vi "Consumer.vi"(8 "error in (no error)":errorcluster, 9 "Data":variant, 10 "Case ID":string, 11 "uService Template in":refnum<class "Father of all uServices.lvclass">) -> (0 "error out":errorcluster, 3 "uService Template out":refnum<class "Father of all uServices.lvclass">)   [LabVIEW 2026, in "TALOS.lvlib" / "Father of all uServices.lvlib" / "Father of all uServices.lvclass"]
uses:
  Father of all uServices.lvclass
  Father of all uServices.lvclass/Father of all uServices.ctl
  Ancestor/Ancestor/Ancestor.lvclass/Ancestor.ctl
  Classes/Log/Log.lvclass/Log.ctl
  45abb896-52c1-49c5-8199-1eb3a3dabe5e.vi
  <vilib>/AdvancedString/1D String Array to Delimited String (string).vi
  <vilib>/AdvancedString/Delimited String to 1D String Array.vi
  <vilib>/AdvancedString/Delimited String to 1D String Array (string).vi
  Support VIs/Generate Error.vi
  Classes/Log/Write.vi
  FGV/Error Memory/Get Error Description.vi
  Support VIs/Get PC name.vi
  Ancestor/Ancestor/Read ID.vi
  Support VIs/Date n Time.vi
  FGV/Error Memory/Error Memory Core.vi
  Support VIs/Circus Root Path.vi
  FGV/Error Memory/Error Crt Lvl checker.vi
  FGV/Error Memory/Error Memory Core.vi/40c8088d-b597-4017-91af-faa98e00292e.vi
  FGV/Error Memory/Error Memory Core.vi/d4a3ab98-063c-4e44-b43d-fbdcfe6c2be2.vi
  <vilib>/Utility/LVClass/Get LV Class Name.vi
  Support VIs/Global Constants.vi
  Support VIs/Global Memory.vi
  Support VIs/Is in Packed Library.vi
  Support VIs/TALOS Root path.vi
  Support VIs/Read CSV worksheet.vi
  <vilib>/Utility/error.llb/General Error Handler.vi
  <vilib>/Utility/config.llb/Open Config Data.vi
  <vilib>/Utility/config.llb/Get Section Names.vi
  <vilib>/Utility/config.llb/Get Key Names.vi
  <vilib>/Utility/config.llb/Read Key.vi
  <vilib>/Utility/config.llb/Read Key (String).vi
  <vilib>/Utility/config.llb/Close Config Data.vi
  Classes/Log/Rotate.vi
  <vilib>/Comparison/Equal/Equal Functor/Equal Functor.lvclass
  Ancestor/Ancestor/Ancestor.lvclass
  TALOS.lvlib
  Classes/Log/Log.lvclass
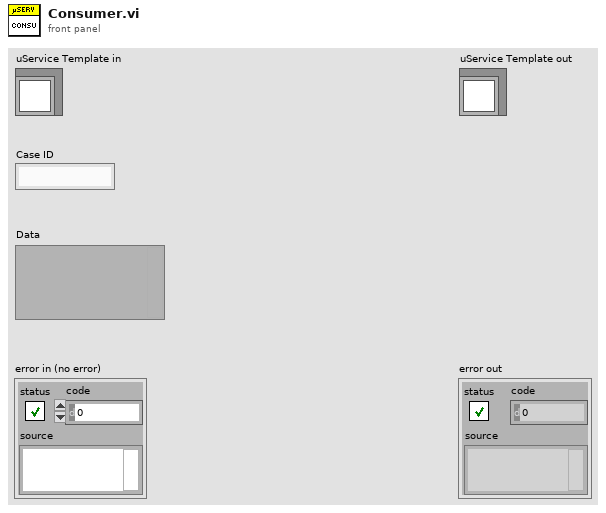
[diagram p1: front panel]
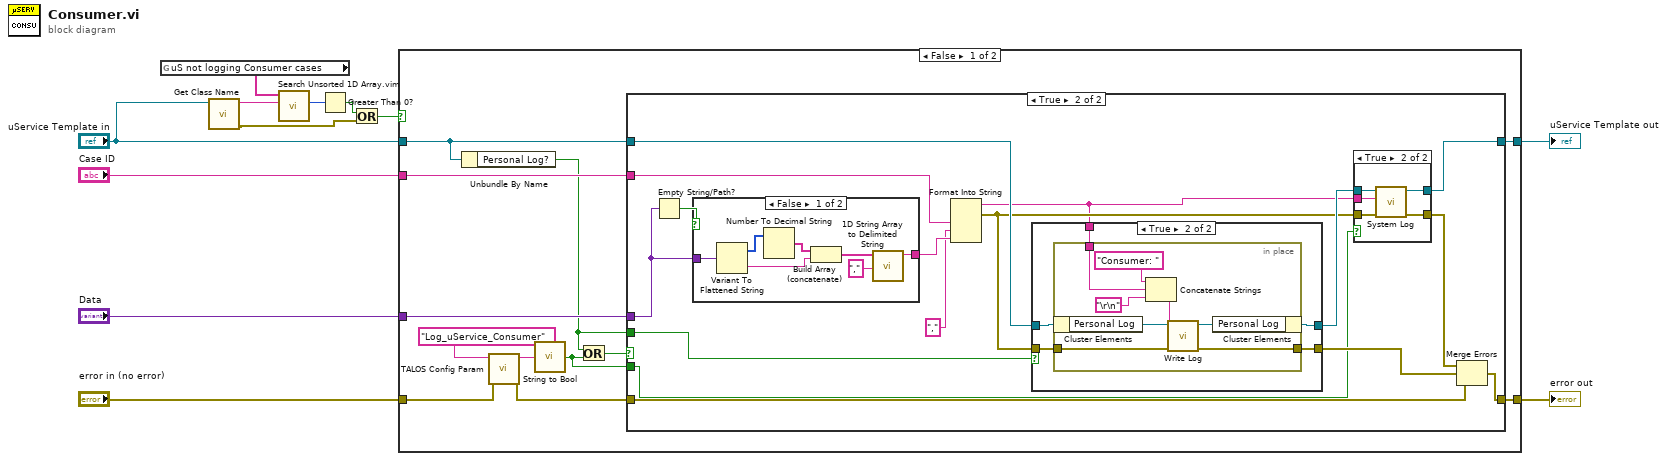
[diagram p0: block diagram]
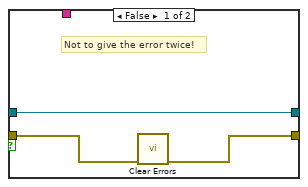
[diagram p4: hidden frame]
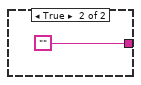
[diagram p5: hidden frame]
diagram:
  n1 = global read "Global Constants.vi" "uS not logging Consumer cases"() -> (w4:string[])
  n2 = call "Get Class Name.vi"("object"="uService Template in") -> ("error out"=w2:errorcluster, "Class Name"=w3:string)  [unwired: 9 in]
  n3 = call "Search Unsorted 1D Array.vim"("element"=w3, "unsorted 1D array"=w4) -> ("index of element"=w6:i32)  [unwired: 9 in]
  n4 = Greater Than 0?(x=w6) -> (x > 0?=w5:bool)
  n5 = Or(x=w5, y=w2) -> (x .or. y?=w1:bool)
  n6 = case shown="False" w1 {
    tunnel: "error in (no error)" -> [w17 w74]
    tunnel: [w24 w74] -> w11
    tunnel: [w23 w75] -> w10
    tunnel: "Case ID" -> [w22 _]
    tunnel: "Data" -> [w21 _]
    tunnel: "uService Template in" -> [w15 w75]
    frame False {
      n7 = Unbundle By Name(w15) -> ("Personal Log?"=w14:bool)
      n8 = call "TALOS Config Param.vi"("error in (no error)"=w17, "Parameter Name"="Log_uService_Consumer") -> ("error out"=w18:errorcluster, "Output"=w20:string)  [unwired: 8 in]
      n9 = call "String to Bool.vi"("String"=w20) -> ("Boolean"=w13:bool)
      n10 = Or(x=w14, y=w13) -> (x .or. y?=w16:bool)
      n11 = case shown="True" w16 {
        tunnel: [w26 w42] -> w24
        tunnel: [w25 w41] -> w23
        tunnel: w22 -> [_ w40]
        tunnel: w21 -> [_ w39]
        tunnel: w15 -> [w25 w31]
        tunnel: w18 -> [w26 w35]
        tunnel: w14 -> [_ w28]
        tunnel: w13 -> [_ w27]
        frame False {
        }
        frame True {
          n12 = Empty String/Path?(string/path=w39) -> (empty?=w38:bool)
          n13 = case shown="False" w38 {
            tunnel: w39 -> [w72 _]
            tunnel: [w66 ""] -> w37
            frame False {
              n14 = Variant To Flattened String(Variant=w72) -> (data string=w68:string, 1:w71:i16[])
              n15 = Number To Decimal String(number=w71) -> (decimal integer string=w69:string[])  [unwired: 1 in]
              n16 = Build Array (concatenate)(w69, w68) -> (w67:string[])
              n17 = call-poly <vilib>:"1D String Array to Delimited String.vi"("delimiter"=",", "string array"=w67) -> ("delimited string"=w66:string)  [unwired: 9 in]
            }
            frame True {
            }
          }
          n18 = Format Into String(w40, "," ("input 2"), w37) -> (resulting string=w29:string, error out=w30:errorcluster)  [unwired: 3 in]
          n19 = case shown="True" w28 {
            tunnel: [w50 w57] -> w33
            tunnel: [w52 w56] -> w32
            tunnel: w31 -> [w52 w55]
            tunnel: w30 -> [w51 w54]
            tunnel: w29 -> [_ w53]
            frame False {
              # "Not to give the error twice!"
              n20 = call <vilib>:"Clear Errors.vi"("error in (no error)"=w51) -> ("error out"=w50:errorcluster)  [unwired: 5 in, 1 out]
            }
            frame True {
              n21 = in-place {
                in-place-border: [w65] -> w57
                in-place-border: w54 -> [w62]
                in-place-border: w53 -> [w61]
                n22 = in-place-cluster #1(w55) -> ("Personal Log"=w64:refnum<class "Log.lvclass">)
                n23 = Concatenate Strings("Consumer: " ("string"), w61, "\r\n") -> (w60:string)
                n24 = call "Write Log.vi"("error in (no error)"=w62, "Text"=w60, "Log in"=w64) -> ("error out"=w65:errorcluster, "Log out"=w63:refnum<class "Log.lvclass">)  [unwired: 7 in]
                n25 = in-place-cluster #1("Personal Log"=w63) -> (w56:refnum<class "Father of all uServices.lvclass">)
              }
            }
          }
          n26 = case shown="True" w27 {
            tunnel: [w44 w49] -> w41
            tunnel: [w43 w48] -> w34
            tunnel: w32 -> [w44 w47]
            tunnel: w30 -> [w43 w46]
            tunnel: w29 -> [_ w45]
            frame False {
            }
            frame True {
              n27 = call "System Log.vi"("error in (no error)"=w46, "Text to log"=w45, "uService Template in"=w47) -> ("error out"=w48:errorcluster, "uService Template out"=w49:refnum<class "Father of all uServices.lvclass">)  [unwired: 7 in]
            }
          }
          n28 = Merge Errors(w34, w33, w35) -> (w42:errorcluster)
        }
      }
    }
    frame True {
    }
  }
  "error out" <- w11
  "uService Template out" <- w10
